vi "송신_멀티캐스트.vi"() -> ()   [LabVIEW 2023]
uses:
  <vilib>/Analysis/NI_AALBase.lvlib
  <vilib>/Utility/tcp.llb/UDP Multicast Write-Only Open.vi
panel:
  in  "Stop Button":bool=TRUE
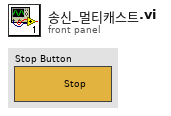
[diagram p1: front panel]
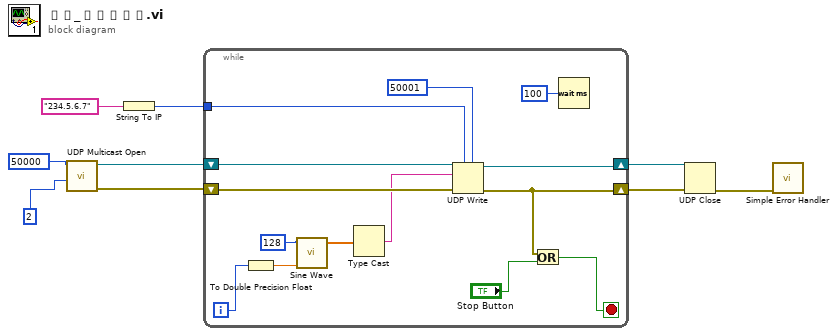
[diagram p0: block diagram]
diagram:
  n1 = call-poly <vilib>:"UDP Multicast Open.vi"("time-to-live (1)"=u16 2, "port"=u16 50000) -> ("error out"=w9:errorcluster, "connection ID"=w7:refnum<k16>)  [unwired: 8 in]
  n2 = String To IP(1:"234.5.6.7" ("Target IP")) -> (0:w5:u32)
  n3 = while {
    shift-right: [w21] -> w6
    shift-left: w7 -> [w22]
    shift-right: [w16] -> w8
    shift-left: w9 -> [w23]
    tunnel: w5 -> [w19]
    i -> [w14]
    stop <- w17 stop-if-true
    n4 = To Double Precision Float(number=w14) -> (double precision float=w13:dbl)
    n5 = call <vilib>:"Sine Wave.vi"("samples"=128, "phase in"=w13) -> ("sine wave"=w12:dbl[])  [unwired: 3 in, 2 out]
    n6 = Type Cast(x=w12) -> (*(type *) &x=w11:string)  [unwired: 1 in]
    n7 = UDP Write(address=w19, port or service name=u16 50001, connection ID=w22, data in=w11, 8:w23) -> (error out=w16:errorcluster, 3:w21:refnum<k16>)  [unwired: 1 in]
    n8 = Or(x=w16, y="Stop Button") -> (x .or. y?=w17:bool)
    n9 = Wait (ms)(milliseconds to wait=u32 100) -> ()  [unwired: 1 out]
  }
  n10 = UDP Close(connection ID=w6, 8:w8) -> (error out=w2:errorcluster)  [unwired: 1 out]
  n11 = call <vilib>:"Simple Error Handler.vi"("error in (no error)"=w2) -> ()  [unwired: 4 in, 5 out]
